vi "PositionNetTrainer.vi"() -> ()   [LabVIEW 2016]
uses:
  <vilib>/Analysis/baseanly.llb/A x Vector.vi
  <vilib>/Analysis/baseanly.llb/Vector x A.vi
  <vilib>/Analysis/baseanly.llb/Real Outer Product.vi
  <vilib>/Analysis/Matrix/Numeric/Multiply/Multiply - RM,R.vi
  <vilib>/Analysis/Matrix/Numeric/Subtract/Subtract - RM,RM.vi
  <vilib>/Analysis/NI_AALBase.lvlib
  <vilib>/Analysis/Matrix/NI_Matrix.lvlib
panel:
  out "Numeric":dbl
  out "W1_new":dbl[][](array[numeric])
  out "W0_new":dbl[][](array[numeric])
  out "J(W0)":dbl[][](array[numeric])
  out "J(W1)":dbl[][](array[numeric])
  out "firstclctn":dbl[](array[numeric])
  out "(yN-t)":dbl[](array[numeric])
  out "delta_N":dbl[](array[numeric])
  out "W_N":dbl[][](array[numeric])
  out "firstclctn.*yN(1-yN)":dbl[](array[numeric])
  out "firstclctn.*yN":dbl[](array[numeric])
  out "y_j":dbl[](array[numeric])
  out "net_j":dbl[](array[numeric])
  out "Input":dbl[](array[numeric])
  out "Weight_j":dbl[][](array[numeric])
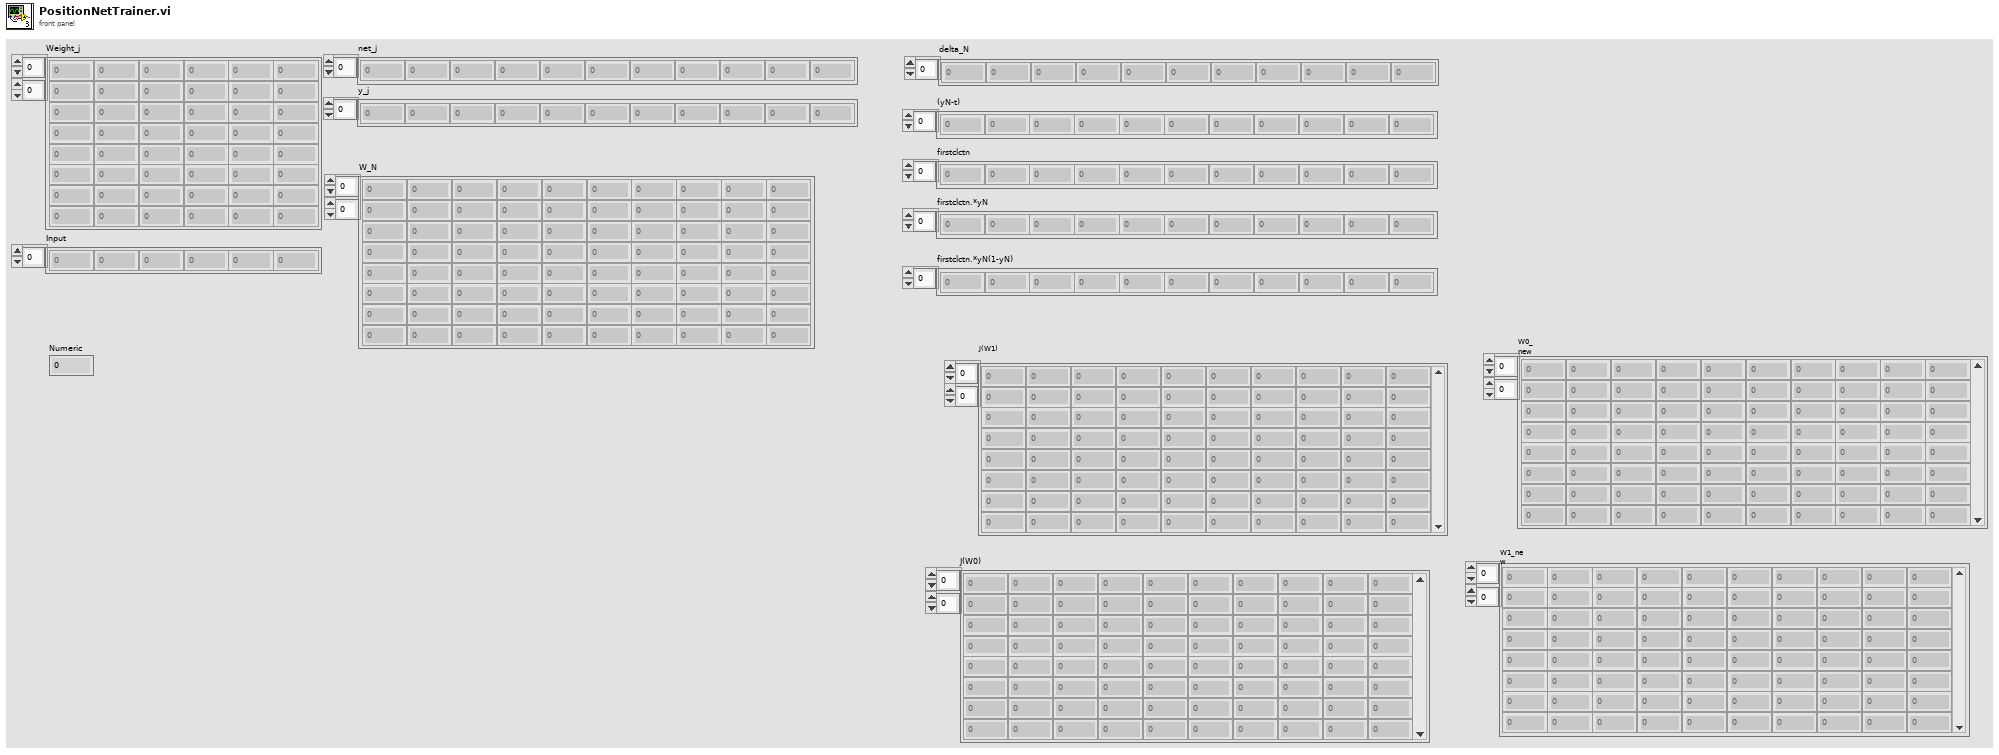
[diagram p1: front panel]
types:
  T1 = typedef "NI_Matrix.lvlib/RealMatrix.ctl" = dbl[][]
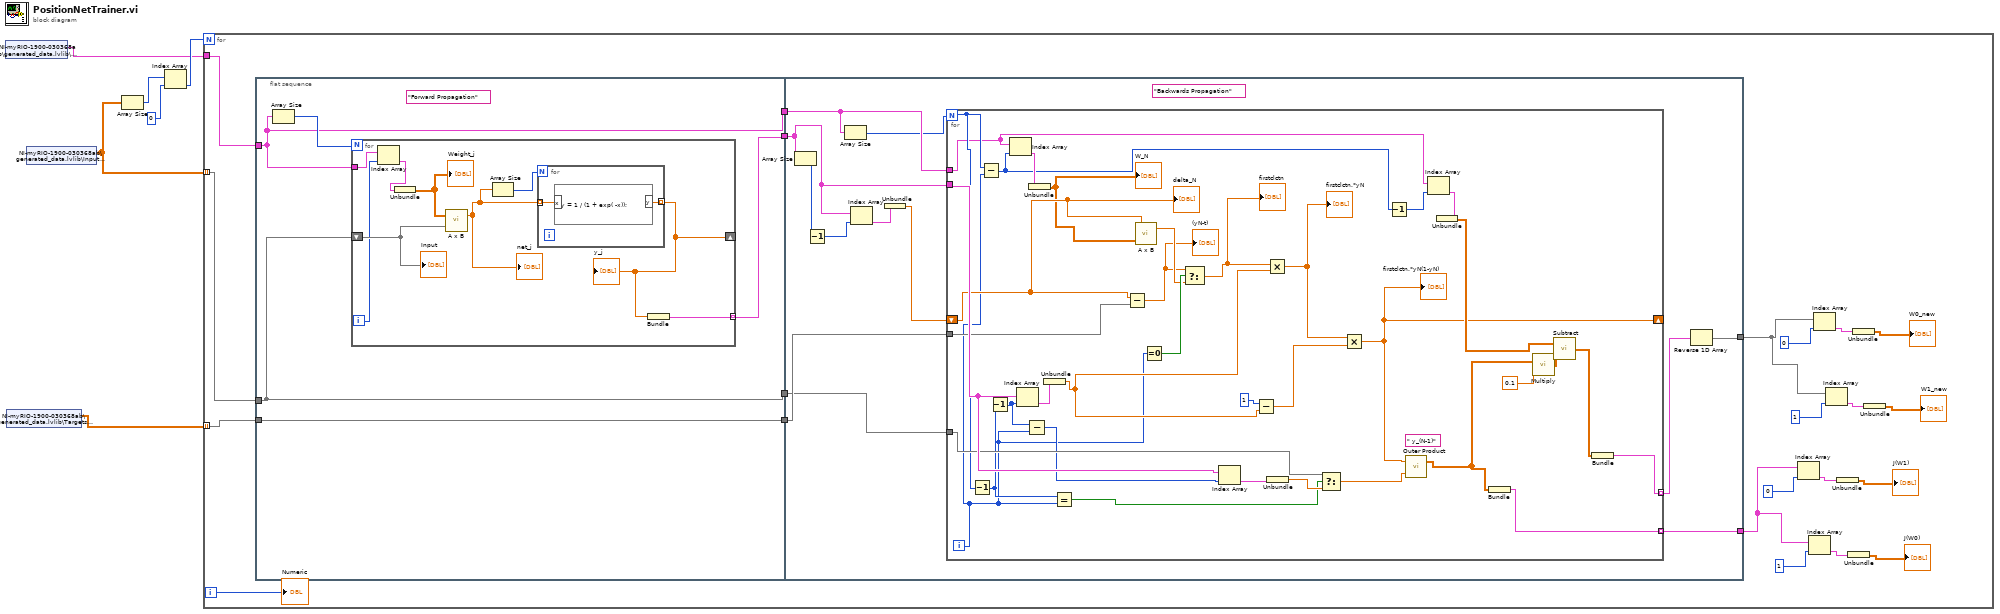
[diagram p0: block diagram]
diagram:
  n1 = shared-variable "NI-myRIO-1900-030368ab\\generated_data.lvlib\\Weights"() -> (w1:cluster{dbl[][]}[])  [unwired: 1 in, 1 out]
  n2 = shared-variable "NI-myRIO-1900-030368ab\\generated_data.lvlib\\Targets_OH"() -> (w6:dbl[][])  [unwired: 1 in, 1 out]
  n3 = shared-variable "NI-myRIO-1900-030368ab\\generated_data.lvlib\\Input Data"() -> (w5:dbl[][])  [unwired: 1 in, 1 out]
  n4 = Array Size(array=w5) -> (size(s)=w4:i32[])
  n5 = Index Array(array=w4, index=0) -> (element=w2:i32)
  n6 = for {
    N: w2 -> [_]
    tunnel: w5 -> [w28] mode=indexing
    tunnel: w6 -> [w26] mode=indexing
    tunnel: w1 -> [w9]
    i -> [w8]
    n7 = flat-sequence {
      tunnel: w9 -> [w31]
      tunnel: w28 -> [w30]
      tunnel: [w32] -> w27
      tunnel: w26 -> [w32]
      tunnel: [w29] -> w25
      tunnel: [w31] -> w24
      tunnel: [w30] -> w23
      tunnel: w27 -> [w49]
      tunnel: w25 -> [w52]
      tunnel: w24 -> [w53]
      tunnel: w23 -> [w48]
      tunnel: [w45] -> w16
      tunnel: [w47] -> w7
      frame #0 {
        (unwired) "Forward Propagation"
        n8 = Array Size(array=w31) -> (size(s)=w33:i32)
        n9 = for {
          N: w33 -> [_]
          tunnel: w31 -> [w36]
          shift-right: [w39] -> _
          shift-left: w30 -> [w40]
          tunnel: [w34] -> w29 mode=indexing
          i -> [w37]
          n10 = Index Array(array=w36, index=w37) -> (element=w35:cluster{dbl[][]})
          n11 = Unbundle(w35) -> (w42:dbl[][])
          "Weight_j" <- w42
          n12 = call-poly <vilib>:"A x B.vi"("Vector"=w40, "A"=w42) -> ("A x Vector"=w38:dbl[])  [unwired: 1 out]
          "net_j" <- w38
          n13 = Array Size(array=w38) -> (size(s)=w41:i32)
          n14 = for {
            N: w41 -> [_]
            tunnel: w38 -> [w44] mode=indexing
            tunnel: [w43] -> w39 mode=indexing
            n15 = formula code="y = 1 / (1 + exp( -x));"("x"=w44) -> ("y"=w43:dbl)
          }
          "y_j" <- w39
          n16 = Bundle(w39) -> (w34:cluster{dbl[]})  [unwired: 1 in]
          "Input" <- w40
        }
      }
      frame #1 {
        (unwired) "Backwards Propagation"
        n17 = Array Size(array=w52) -> (size(s)=w55:i32)
        n18 = Decrement(x=w55) -> (x-1=w54:i32)
        n19 = Array Size(array=w53) -> (size(s)=w51:i32)
        n20 = Index Array(array=w52, index=w54) -> (element=w56:cluster{dbl[]})
        n21 = Unbundle(w56) -> (w50:dbl[])
        n22 = for {
          N: w51 -> [w72]
          tunnel: w53 -> [w68]
          tunnel: w52 -> [w92]
          tunnel: w48 -> [w91]
          shift-right: [w63] -> _
          shift-left: w50 -> [w80]
          tunnel: w49 -> [w79]
          tunnel: [w58] -> w46 mode=indexing
          tunnel: [w57] -> w45 mode=indexing
          i -> [w71]
          (unwired) " y_(N-1)"
          n23 = Decrement(x=w72) -> (x-1=w73:i32)
          n24 = Subtract(x=w72, y=w71) -> (x-y=w70:i32)
          n25 = Decrement(x=w73) -> (x-1=w82:i32)
          n26 = Index Array(array=w68, index=w70) -> (element=w90:cluster{dbl[][]})
          n27 = Index Array(array=w92, index=w82) -> (element=w87:cluster{dbl[]})
          n28 = Subtract(x=w82, y=w71) -> (x-y=w81:i32)
          n29 = Unbundle(w90) -> (w74:dbl[][])
          "W_N" <- w74
          n30 = Unbundle(w87) -> (w86:dbl[])
          n31 = Equal?(x=w73, y=w71) -> (x = y?=w83:bool)
          n32 = Subtract(x=w80, y=w79) -> (x-y=w76:dbl[])
          "(yN-t)" <- w76
          n33 = call-poly <vilib>:"A x B.vi"("Matrix A"=w74, "Vector V'"=w80) -> ("V' x A"=w77:dbl[])  [unwired: 1 out]
          n34 = Equal To 0?(x=w71) -> (x = 0?=w78:bool)
          n35 = Select(t=w76, s=w78, f=w77) -> (s? t:f=w75:dbl[])
          "firstclctn" <- w75
          n36 = Index Array(array=w92, index=w81) -> (element=w89:cluster{dbl[]})
          n37 = Subtract(x=1, y=w86) -> (x-y=w85:dbl[])
          n38 = Multiply(x=w75, y=w86) -> (x*y=w88:dbl[])
          "firstclctn.*yN" <- w88
          n39 = Unbundle(w89) -> (w84:dbl[])
          n40 = Select(t=w91, s=w83, f=w84) -> (s? t:f=w64:dbl[])
          n41 = Multiply(x=w88, y=w85) -> (x*y=w63:dbl[])
          "firstclctn.*yN(1-yN)" <- w63
          n42 = Decrement(x=w70) -> (x-1=w69:i32)
          n43 = call-poly <vilib>:"Outer Product.vi"("Y Vector"=w64, "X Vector"=w63) -> ("Outer Product"=w62:T1)  [unwired: 1 out]
          n44 = Index Array(array=w68, index=w69) -> (element=w67:cluster{dbl[][]})
          n45 = Unbundle(w67) -> (w65:dbl[][])
          n46 = Bundle("Outer Product"=w62) -> (w57:cluster{"Outer Product":T1})  [unwired: 1 in]
          n47 = call-poly <vilib>:"Multiply.vi"("Real Scalar c"=0.1, "Real Matrix A"=w62) -> ("A * c"=w60:T1)
          n48 = call-poly <vilib>:"Subtract.vi"("Real Matrix B"=w60, "Real Matrix A"=w65) -> ("A - B"=w66:T1)
          n49 = Bundle("A - B"=w66) -> (w58:cluster{"A - B":T1})  [unwired: 1 in]
          "delta_N" <- w80
        }
        n50 = Reverse 1D Array(array=w46) -> (reversed array=w47:cluster{"A - B":T1}[])
      }
    }
    n51 = Index Array(array=w16, index=0) -> (element=w22:cluster{"Outer Product":T1})
    n52 = Index Array(array=w16, index=1) -> (element=w19:cluster{"Outer Product":T1})
    n53 = Index Array(array=w7, index=0) -> (element=w15:cluster{"A - B":T1})
    n54 = Index Array(array=w7, index=1) -> (element=w12:cluster{"A - B":T1})
    n55 = Unbundle(w22) -> ("Outer Product"=→"J(W1)":T1)
    n56 = Unbundle(w19) -> ("Outer Product"=→"J(W0)":T1)
    n57 = Unbundle(w15) -> ("A - B"=→"W0_new":T1)
    n58 = Unbundle(w12) -> ("A - B"=→"W1_new":T1)
    "Numeric" <- w8
  }
